vi "EtherNet_IP Test VI.vi"() -> ()   [LabVIEW 2020, in "EtherNet_IP_Lib.lvlib"]
uses:
  EtherNet_IP_Lib.lvlib
panel:
  out "ms for Each Scan":u32
  in  "No of Elements":u8
  in  "Offset(N7:?)":u8
  out "Data Error":bool
  out "Data Out":u16[](array[numeric])=[29379, 41832, 41776, 41777, 41778, 41779]
  out "error out":errorcluster
  in  "Exit":bool
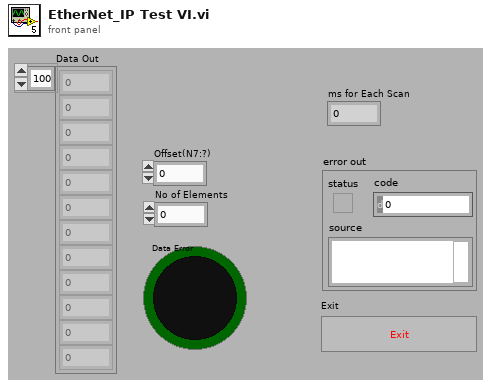
[diagram p1: front panel]
types:
  T1 = cluster{"TCP Connection":refnum<k5>, "Session":u8[], "EtherNet/IP Device Address":string}
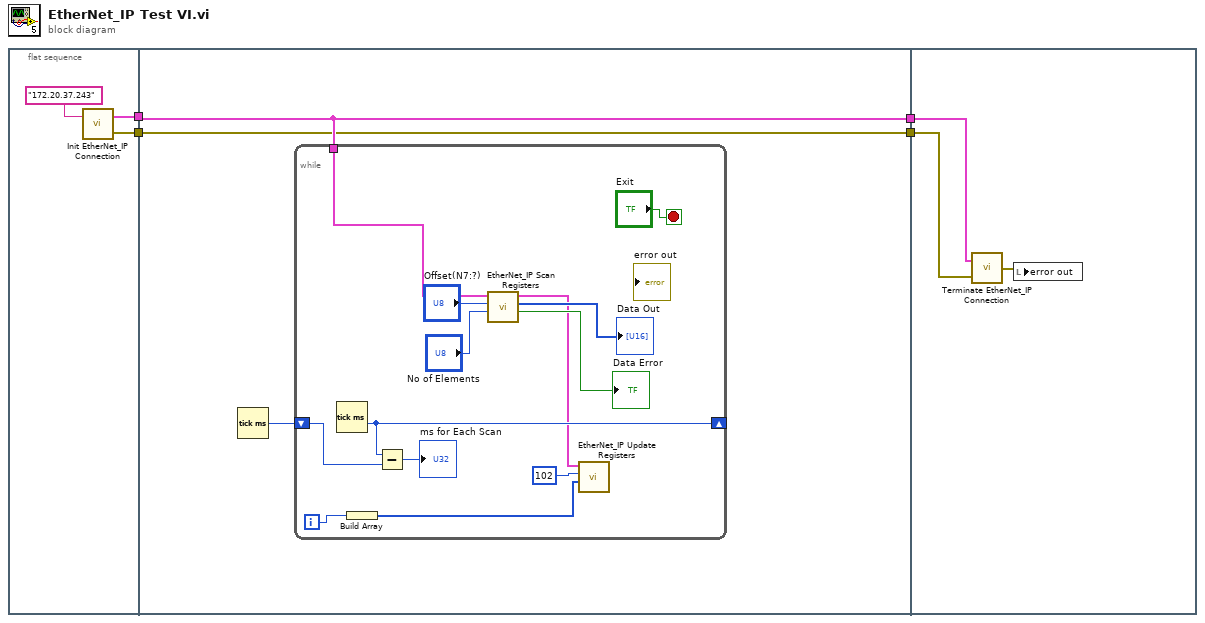
[diagram p0: block diagram]
diagram:
  n1 = flat-sequence {
    tunnel: [w6] -> w4
    tunnel: [w5] -> w3
    tunnel: w4 -> [w10]
    tunnel: w3 -> [w9]
    tunnel: [w10] -> w2
    tunnel: [w9] -> w1
    tunnel: w2 -> [w26]
    tunnel: w1 -> [w25]
    frame #0 {
      n2 = call "Init EtherNet_IP Connection.vi"("EtherNet/IP Device Address"="172.20.37.243") -> ("error out"=w5:errorcluster, "Connection Cluster"=w6:T1)  [unwired: 1 in]
    }
    frame #1 {
      n3 = Tick Count (ms)() -> (millisecond timer value=w8:u32)
      n4 = while {
        tunnel: w10 -> [w15]
        shift-right: [w18] -> _
        shift-left: w8 -> [w17]
        i -> [w12]
        stop <- "Exit" stop-if-true
        n5 = Tick Count (ms)() -> (millisecond timer value=w18:u32)
        n6 = Build Array(w12) -> (w11:i32[])
        n7 = Subtract(x=w18, y=w17) -> (x-y=→"ms for Each Scan":u32)
        n8 = call "EtherNet_IP Scan Registers.vi"("No of Elements"="No of Elements", "Offset(N7:?)"="Offset(N7:?)", "Connection Cluster"=w15) -> ("Data Error"=→"Data Error":bool, "Registers"=→"Data Out":u16[], "Connection Cluster Out"=w13:T1)  [unwired: 1 in, 1 out]
        n9 = call "EtherNet_IP Update Registers.vi"("Registers"=w11, "Offset(N7:?)"=u8 102, "Connection Cluster"=w13) -> ()  [unwired: 1 in, 3 out]
      }
    }
    frame #2 {
      n10 = call "Terminate EtherNet_IP Connection.vi"("error in"=w25, "Connection Cluster"=w26) -> ("error out"=w24:errorcluster)
      n11 = local write "error out"(w24) -> ()
    }
  }
